vi "micron_ui.vi"() -> ()   [LabVIEW 2014]
uses:
  testing/Trace controls.ctl
  testing/probe_point.ctl
  cancellation/sq_control_params.ctl
  cancellation/decoupled_gain.ctl
  testing/mode_conrols.ctl
  testing/control_selector.ctl
  testing/stimulus.ctl
  testing/injection_point.ctl
  filtering/goal_loop_parms.ctl
  host/network_params.ctl
  cancellation/estimation_controls.ctl
  testing/flag_selector.ctl
  testing/status_flag.ctl
  testing/pose_selector.ctl
  testing/pose_source.ctl
  testing/pose_relative_to.ctl
  testing/log_event.ctl
  <vilib>/Platform/TimedLoop/XDataNode/timing_clust.ctl
  <vilib>/Platform/TimedLoop/XDataNode/nitl_modes.ctl
  <vilib>/Platform/TimedLoop/XDataNode/wakeup.ctl
  testing/ui_override_opts.ctl
  initialization/micron_globals.vi
  <vilib>/Utility/xml.llb/Read From XML File(array).vi
  <vilib>/Utility/xml.llb/Write to XML File(string).vi
  <vilib>/Platform/TimedLoop/XDataNode/XDataNode.xnode
  <vilib>/Platform/TimedLoop/XDataNode/XDNodeRunTimeDep.lvlib
panel:
  in  "Tab Control":T1(tab)
  in  "Goal filter A":T2={"Speedup max"=100.0, "Speedup thresh"=1500.0, "Speedup nonlin"=2.0, "Filters"=[{"Lower Fc"=0.05, "Lower Q"=0.62, "Scale factor"=3.0, "Upper Fc"=2.0, "Upper Q"=0.62, "V limit"=1000.0, "V limit range"=1000.0}, {"Lower Fc"=0.05, "Lower Q"=0.62, "Scale factor"=3.0, "Upper Fc"=2.0, "Upper Q"=0.62, "V limit"=1000.0, "V limit range"=1000.0}]} {"Filters"."V limit range" format="%_3p"; "Filters"."V limit" format="%_3p"; "Filters"."Upper Q" format="%_3f"; "Filters"."Upper Fc" format="%_3p"; "Filters"."Lower Q" format="%_3f"; "Filters"."Scale factor" format="%_3f"; "Filters"."Lower Fc" format="%_3p"; "Speedup nonlin" format="%_3p"; "Speedup thresh" format="%_3p"; "Speedup max" format="%_3p"}
  in  "Goal filter B":T2={"Speedup max"=10.0, "Speedup thresh"=750.0, "Speedup nonlin"=2.0, "Filters"=[{"Lower Fc"=1.5, "Lower Q"=0.62, "Scale factor"=1.0, "Upper Fc"=1.5, "Upper Q"=0.62, "V limit"=1000.0, "V limit range"=0.0}, {"Lower Fc"=1.5, "Lower Q"=0.62, "Scale factor"=1.0, "Upper Fc"=1.5, "Upper Q"=0.62, "V limit"=1000.0, "V limit range"=0.0}]} {"Filters"."V limit range" format="%_3p"; "Filters"."V limit" format="%_3p"; "Filters"."Upper Q" format="%_3f"; "Filters"."Upper Fc" format="%_3p"; "Filters"."Lower Q" format="%_3f"; "Filters"."Scale factor" format="%_3f"; "Filters"."Lower Fc" format="%_3p"; "Speedup nonlin" format="%_3p"; "Speedup thresh" format="%_3p"; "Speedup max" format="%_3p"}
  in  "Transition time":sgl=1.0
  in  "Cancellation":T3={"KP"={"XY"=0.5, "Rxy"=0.5, "Z"=0.2, "Rz"=0.1}, "KI"=0.0, "KD"={"XY"=-0.2, "Rxy"=0.0, "Z"=0.0, "Rz"=0.0}, "Max vel"=13.0, "Max acc"=2.0, "Int error limit"=3.0, "RCM gain"=1.0, "Bypass"=FALSE, "Degraded gain"=0.4} {"Degraded gain" min=0 max=1 step=0.1 format="%#_3p"; "RCM gain" min=0 max=1 step=0.1 format="%#_3p"; "KD"."Rz" min=-1 max=1 step=0.01 format="%#_3p"; "KD"."Rxy" min=-1 max=1 step=0.01 format="%#_3p"; "KD"."Z" min=-1 max=1 step=0.01 format="%#_3p"; "KD"."XY" min=-1 max=1 step=0.01 format="%#_3p"; "KI" min=0 max=1 step=0.01 format="%#_3p"; "KP"."Rz" min=-1 max=1 step=0.01 format="%#_3p"; "KP"."Rxy" min=-1 max=1 step=0.01 format="%#_3p"; "KP"."Z" min=-1 max=1 step=0.01 format="%#_3p"; "KP"."XY" min=-1 max=1 step=0.01 format="%#_3p"; "Max acc" format="%#_3p"}
  in  "Estimation":T5={"Link"={"Measure noise"=[4.0], "Process noise"=[15.0, 1.0], "Alt process noise"=[20.0], "Alt turnoff cycles"=20, "Innovation limit"=[inf], "Residue threshold"=20.0, "Enable"=TRUE}, "Handle"={"Measure noise"=[3.6, 0.00036], "Process noise"=[0.0, 0.0, 0.3, 0.0, 0.0006, 0.3, 1.0, 0.3, 0.3, 1.0], "State limits"=[], "Innovation limit"=[], "Prediction Lookahead"=1.5, "Enable"=TRUE}}
  in  "Manipulator disable":bool
  in  "Network":T6={"Remote Host"="192.168.1.3", "Send Status"=TRUE, "Send Port"=61557, "Recv Commands"=FALSE, "Recv Port"=61557}
  in  "Light enables":bool[](array[boolean])=[TRUE, TRUE, TRUE, TRUE, TRUE, TRUE]
  out "Trace display":T7(graph)
  out "Warning":bool
  out "Error":bool
  out "Status":T8[](array[typedef]) {"Timestamp" format="%<%.3X>T"}
  in  "Reference hold":bool
  in  "Pose selectors":T9[](array[typedef])
  in  "Recenter":bool
  out "RCM limit":bool
  out "Stall":bool[](array[boolean])
  out "Link lengths":sgl[](array[slide]) scale=-1.0..1.0
  out "Saturation":bool
  out "Speedup":sgl(slide) scale=1.0..50.0
  in  "Flag selectors":T12[](array[typedef])
  in  "Averaging":bool
  in  "Reset":bool
  out "Run/stop":bool
  in  "Trigger":bool
  in  "Trigger mode":bool
  in  "Calibration":bool=TRUE
  in  "Parameters":bool=TRUE
  in  "Controls":bool=TRUE
  in  "Load":bool
  in  "Configurations":i32(listbox)
  in  "Save":bool
  in  "Save as":bool
  in  "Config name":string="default"
  in  "Finder":bool=TRUE
  out "Position":sgl[](array[numeric]) format="%9.1f"
  in  "Stimulus":T14={"Type"=enum."Off", "Phase"=0.0, "Amplitude"=[0.0, 200.0, 0.0, 0.0, 0.0, 0.0], "Injection point"=enum."Total pose", "Closed loop"=TRUE, "Offset"=[0.0, 0.0, 0.0, 0.0, 0.0, 0.0], "Tip -> world"=TRUE, "Frequency"=1.0, "Length"=1.0} {"Length" min=0.0 max=100.0 step=100.0 format="%#_4p"; "Frequency" min=0.0 step=100.0 format="%#_4g"; "Offset" format="%#_3p"; "Amplitude" format="%#_3p"; "Phase" min=-180.0 max=360.0 step=100.0 format="%#.2f"}
  in  "Pedal selector":T16[](array[typedef])=[{"Selection"=enum."Right", "Mode"=enum."Never"}, {"Selection"=enum."Left", "Mode"=enum."Toggle"}, {"Selection"=enum."Right", "Mode"=enum."Toggle"}, {"Selection"=enum."Middle", "Mode"=enum."Pulse"}]
  out "Mode controls":T17={"Hold"=FALSE, "Cancellation"=TRUE, "Goal filter"=TRUE, "Trigger"=FALSE}
  in  "Decimate":i32=20 min=1 max=999 step=1
  in  "Trace path":path
  in  "Save trace":bool
  out "2D position":cluster{"X":sgl[], "Y":sgl[]}[](graph)
  in  "Trace controls":T18[](array[typedef])=[{"+ stim"=FALSE, "Relative"=FALSE, "Scale"=enum."1X", "Probe point"=enum."Position (tip)", "XYZ selector"={"Boolean"=FALSE, "Boolean 2"=FALSE, "Boolean 3"=FALSE}, "To tip"=FALSE}, {"+ stim"=FALSE, "Relative"=FALSE, "Scale"=enum."1X", "Probe point"=enum."Position (tip)", "XYZ selector"={"Boolean"=FALSE, "Boolean 2"=FALSE, "Boolean 3"=FALSE}, "To tip"=FALSE}, {"+ stim"=FALSE, "Relative"=FALSE, "Scale"=enum."1X", "Probe point"=enum."Position (tip)", "XYZ selector"={"Boolean"=FALSE, "Boolean 2"=FALSE, "Boolean 3"=FALSE}, "To tip"=FALSE}, {"+ stim"=FALSE, "Relative"=FALSE, "Scale"=enum."1X", "Probe point"=enum."Position (tip)", "XYZ selector"={"Boolean"=FALSE, "Boolean 2"=FALSE, "Boolean 3"=FALSE}, "To tip"=FALSE}]
  in  "stop":bool
  # "m  Micron interface"
  # "Triggering"
  # "One-shot"
  # "Continuous"
  # "Trace Display"
  # "Used for ASAP testing.  Not saved in config."
  # "Configuration Manager"
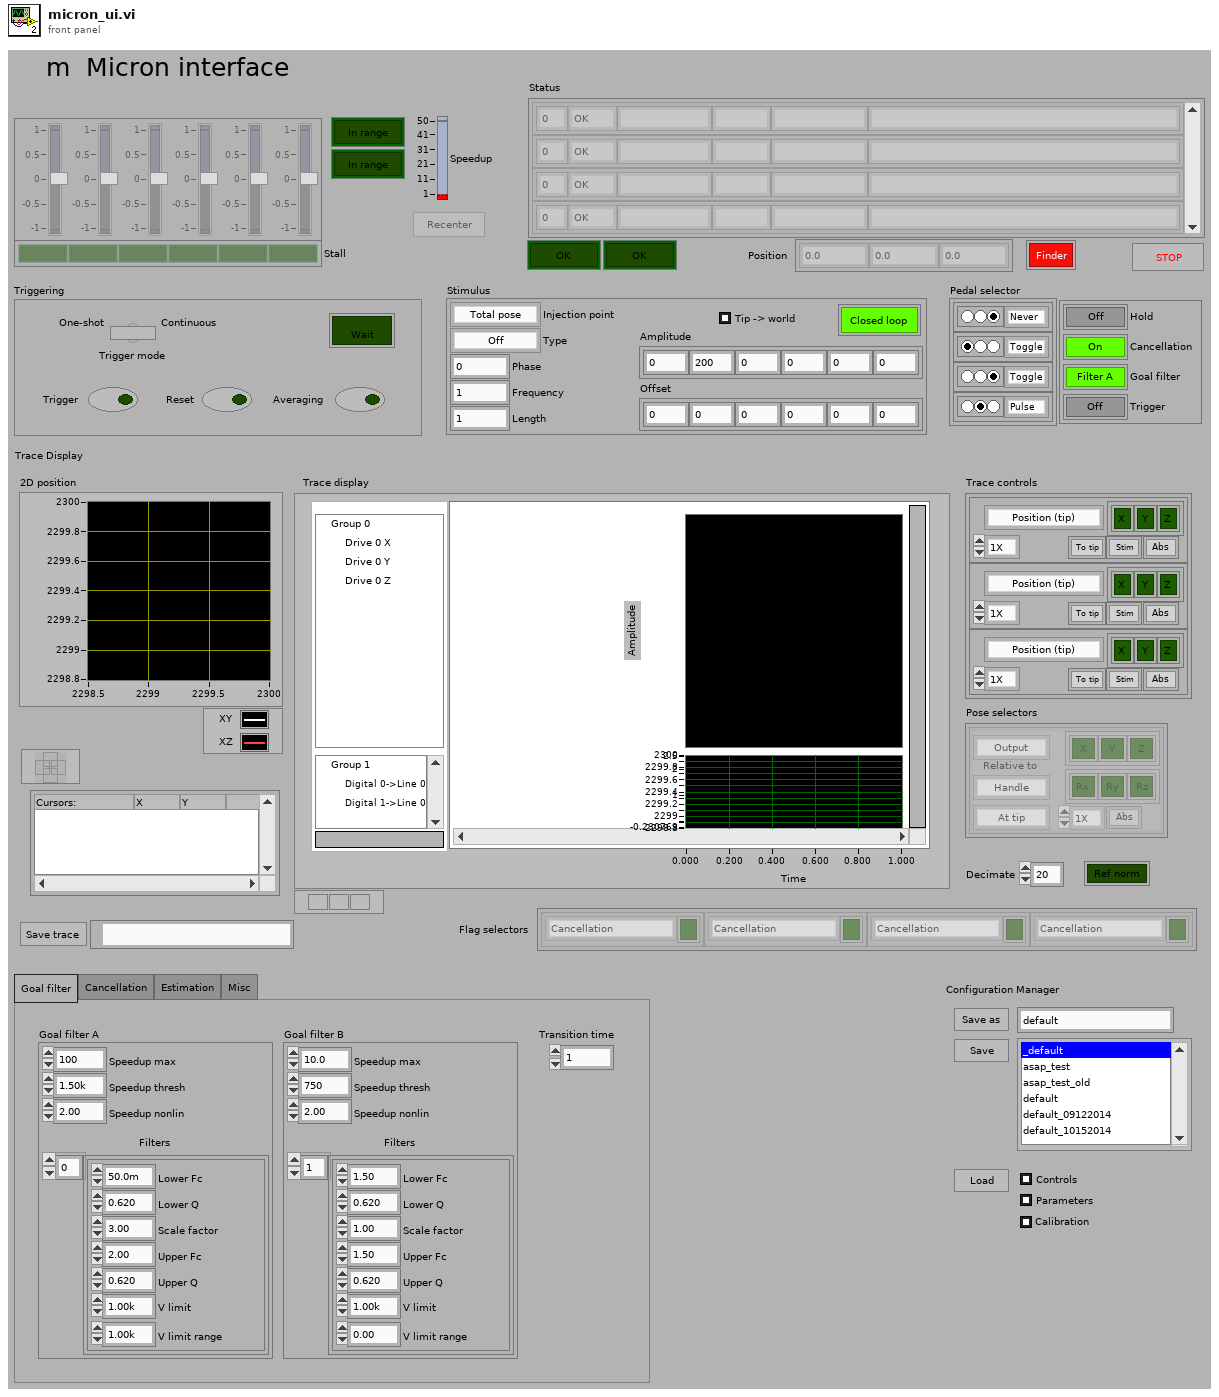
[diagram p1: front panel]
types:
  T1 = enum32{"Goal filter", "Cancellation", "Estimation", "Misc"}
  T2 = typedef "goal_loop_parms.ctl" = cluster{"Speedup max":sgl, "Speedup thresh":sgl, "Speedup nonlin":sgl, "Filters":cluster{"Lower Fc":sgl, "Lower Q":sgl, "Scale factor":sgl, "Upper Fc":sgl, "Upper Q":sgl, "V limit":sgl, "V limit range":sgl}[]}
  T3 = typedef "sq_control_params.ctl" = cluster{"KP":T4, "KI":sgl, "KD":T4, "Max vel":sgl, "Max acc":sgl, "Int error limit":sgl, "RCM gain":sgl, "Bypass":bool, "Degraded gain":sgl}
  T4 = typedef "decoupled_gain.ctl" = cluster{"XY":sgl, "Rxy":sgl, "Z":sgl, "Rz":sgl}
  T5 = typedef "estimation_controls.ctl" = cluster{"Link":cluster{"Measure noise":dbl[], "Process noise":dbl[], "Alt process noise":dbl[], "Alt turnoff cycles":i32, "Innovation limit":dbl[], "Residue threshold":dbl, "Enable":bool}, "Handle":cluster{"Measure noise":dbl[], "Process noise":dbl[], "State limits":dbl[], "Innovation limit":dbl[], "Prediction Lookahead":sgl, "Enable":bool}}
  T6 = typedef "network_params.ctl" = cluster{"Remote Host":string, "Send Status":bool, "Send Port":u16, "Recv Commands":bool, "Recv Port":u16}
  T7 = cluster{"Waveforms out":waveform(sgl)[], "Digital waveforms":digitalwaveform[]}
  T8 = typedef "log_event.ctl" = cluster{"Facility ID":i32, "Severity":enum16{"OK", "Debug", "Warn", "Error"}, "Timestamp":timestamp, "Facility":string, "State":string, "Message":string}
  T9 = typedef "pose_selector.ctl" = cluster{"Scale":enum16{"1X", "10X", "100X", "1KX", "10KX"}, "Source":T10, "XYZ selector":cluster{"Boolean":bool, "Boolean 2":bool, "Boolean 3":bool}, "RPY selector":cluster{"Boolean":bool, "Boolean 2":bool, "Boolean 3":bool}, "Relative to":T11, "Relative":bool, "Translate":enum16{"At tip", "At RCM", "At KC", "At origin"}}
  T10 = typedef "pose_source.ctl" = enum16{"Output", "Handle", "Handle KF", "Goal", "Absolute"}
  T11 = typedef "pose_relative_to.ctl" = enum16{"Output", "Handle", "Handle KF", "Goal", "Absolute", "Trace start"}
  T12 = typedef "flag_selector.ctl" = cluster{"Flag":T13, "Select":bool}
  T13 = typedef "status_flag.ctl" = enum16{"Cancellation", "Goal filter", "Valid position", "Goal saturation tip", "Goal saturation RCM", "Goal circle saturation", "Position saturation", "Output saturation", "Acceleration limiting", "Finished late", "Stimulus increasing", "Integral error saturation", "Velocity limiting", "Log warning", "Log error", "Link KF degraded"}
  T14 = typedef "stimulus.ctl" = cluster{"Type":enum16{"Off", "Step", "Sine", "Triangle", "Arbitrary"}, "Phase":dbl, "Amplitude":sgl[], "Injection point":T15, "Closed loop":bool, "Offset":sgl[], "Tip -> world":bool, "Frequency":dbl, "Length":dbl}
  T15 = typedef "injection_point.ctl" = enum16{"Total pose", "V limiter", "Goal ", "Link position", "KF link position", "Inverse kin", "Link goal", "Link error", "Controller", "Output", "Drive", "Light"}
  T16 = typedef "control_selector.ctl" = cluster{"Selection":enum32{"No Selection", "Left", "Middle", "Right"}, "Mode":enum16{"Up", "Down", "Toggle", "Pulse", "Always", "Never"}}
  T17 = typedef "mode_conrols.ctl" = cluster{"Hold":bool, "Cancellation":bool, "Goal filter":bool, "Trigger":bool}
  T18 = typedef "Trace controls.ctl" = cluster{"+ stim":bool, "Relative":bool, "Scale":enum16{"1X", "10X", "100X", "1KX", "10KX"}, "Probe point":T19, "XYZ selector":cluster{"Boolean":bool, "Boolean 2":bool, "Boolean 3":bool}, "To tip":bool}
  T19 = typedef "probe_point.ctl" = enum16{"Position (tip)", "Position (RCM)", "Null pos (tip)", "Null pos (RCM)", "V limiter (tip)", "V Limiter (RCM)", "Goal filter (tip)", "Goal filter (RCM)", "Goal force (tip)", "Goal force (RCM)", "Goal (tip)", "Goal (RCM)", "Link pos 0", "Link pos 1", "KF link pos 0", "KF link pos 1", "Link rate 0", "Link rate 1", "Link residue 0", "Link residue 1", "Link goal 0", "Link goal 1", "Rate limit 0", "Rate limit 1", "Link error 0", "Link error 1", "Controller 0", "Controller 1", "Output 0", "Output 1", "Drive 0", "Drive 1", "Stimulus 0", "Stimulus 1", "Trace data 0", "Trace data 1", "Analog data 0", "Analog data 1", "Status flags", "Light 0", "Light 1", "Light 2", "Light 3", "Light 4", "Light 5", "Goal origin", "Goal rotation 0", "Goal rotation 1", "Goal rotation 2", "Output origin", "Output rotation 0", "Output rotation 1", "Output rotation 2", "Handle origin", "Handle rotation 0", "Handle rotation 1", "Handle rotation 2", "Handle position", "Handle velocity", "Handle acceleration", "Handle angles", "Handle angle rates", "Handle pos residue", "Handle angle residue", "Trace length"}
  T20 = typedef "XDNodeRunTimeDep.lvlib/timing_clust.ctl" = cluster{"Expected End [f-1]":u64, "Actual End [f-1]":u64, "Finished Late? [f-1]":bool, "Expected End [i-1]":u64, "Actual End [i-1]":u64, "Finished Late? [i-1]":bool, "Expected Start [i]":u64, "Actual Start [i]":u64, "Expected Start [f]":u64, "Actual Start [f]":u64, "Source Name":string, "Structure Name":string, "Period":i64, "Deadline":i64, "Offset":i64, "Start":i64, "Priority":i32, "Timeout":i32, "Mode":T21, "Wakeup Reason":T22, "Error":errorcluster, "Source Type":string, "Secondary Source Type":string, "Global End Time":u64, "Global Start Time":u64, "Frame Duration":u64, "Iteration Duration":u64, "Assigned CPU":i32, "I/O Scan Engine Mode":u32}
  T21 = typedef "XDNodeRunTimeDep.lvlib/nitl_modes.ctl" = enum32{"No Change", "Process missed periods, maintain original phase", "Discard missed periods, maintain original phase", "Process missed periods, ignore original phase", "Discard missed periods, ignore original phase"}
  T22 = typedef "XDNodeRunTimeDep.lvlib/wakeup.ctl" = enum32{"Normal", "Aborted", "Asynchronous wakeup", "Timing source error", "Timed loop error", "Timeout"}
  T23 = typedef "micron_config.ctl" = cluster{"rt fifo":refnum<k33>, "Analog output task":refnum<k21>, "Analog output task 2":refnum<k21>, "Stimulus AO task":refnum<k21>, "Low-rate AIN task":refnum<k21>, "Pedal out task":refnum<k21>, "Pedal in task":refnum<k21>, "Loop timing source":string, "Relay out task":refnum<k21>, "Send UDP Conn":refnum<k16>, "Recv UDP Conn":refnum<k16>, "Host Addr":u32, "I2C interface":T24, "trace_start notifier":refnum<notifier>, "trace_done notifier":refnum<notifier>, "ASAP FIFO":refnum<k33>}
  T24 = typedef "i2c_interface.ctl" = cluster{"FPGA VI Reference":T25}
  T25 = typedef "fpga_reference.ctl" = refnum<k20>
  T26 = typedef "configuration.ctl" = cluster{"Calibration data":T27, "Block size":i32, "Tasks":cluster{"Analog Input":refnum<k21>, "Counters":refnum<k21>[], "Digital out":refnum<k21>}, "Light enables":bool[]}
  T27 = typedef "asap_calibration.ctl" = cluster{"T1":T28, "K1":T28, "T2":T28, "K2":T28, "Sensor LUT":sgl[][][][]}
  T28 = typedef "NI_Matrix.lvlib/RealMatrix.ctl" = dbl[][]
  T29 = enum8{"Enabled", "Disabled", "Disabled and Grayed Out"}
  T30 = typedef "Micron params.ctl" = cluster{"Stimulus":T14, "Goal Filter A":T2, "Mode controls":T17, "Manipulator type":enum16{"Current piezo", "Voltage piezo"}, "Manipulator calibration":T31, "Network":T6, "Goal Filter B":T2, "Cancellation":T3, "Transition time":sgl, "Estimation":T5}
  T31 = typedef "manipulator_cal.ctl" = cluster{"Tool offsets":sgl[][], "Handle light calibration":T32, "Base pivots":sgl[][], "Output pivots":sgl[][], "Length center":sgl, "Workspace height":sgl[], "Workspace diameter":sgl[], "Stack travel":sgl, "Saturation pos":sgl, "Inverse filters":cluster{"filter structure":enum32{"IIR 2nd Order", "IIR 4th Order"}, "Reverse Coefficients":dbl[], "Forward Coefficients":dbl[]}[], "Strut length":sgl, "Tip light calibration":T32}
  T32 = typedef "probe_calibration.ctl" = sgl[][]
  T33 = typedef "ui_override_opts.ctl" = cluster{"Triggering":bool, "Parameters":bool, "Stimulus":bool, "Calibration":bool, "Modes":bool}
  T34 = enum16{"Up", "Down", "Toggle", "Pulse", "Always", "Never"}
  T35 = cluster{"Finder":bool, "Trigger mode":bool, "Pedal selector":T16[], "Decimate":i32, "Trace controls":T18[], "Flag selectors":T12[], "Pose selectors":T9[]}
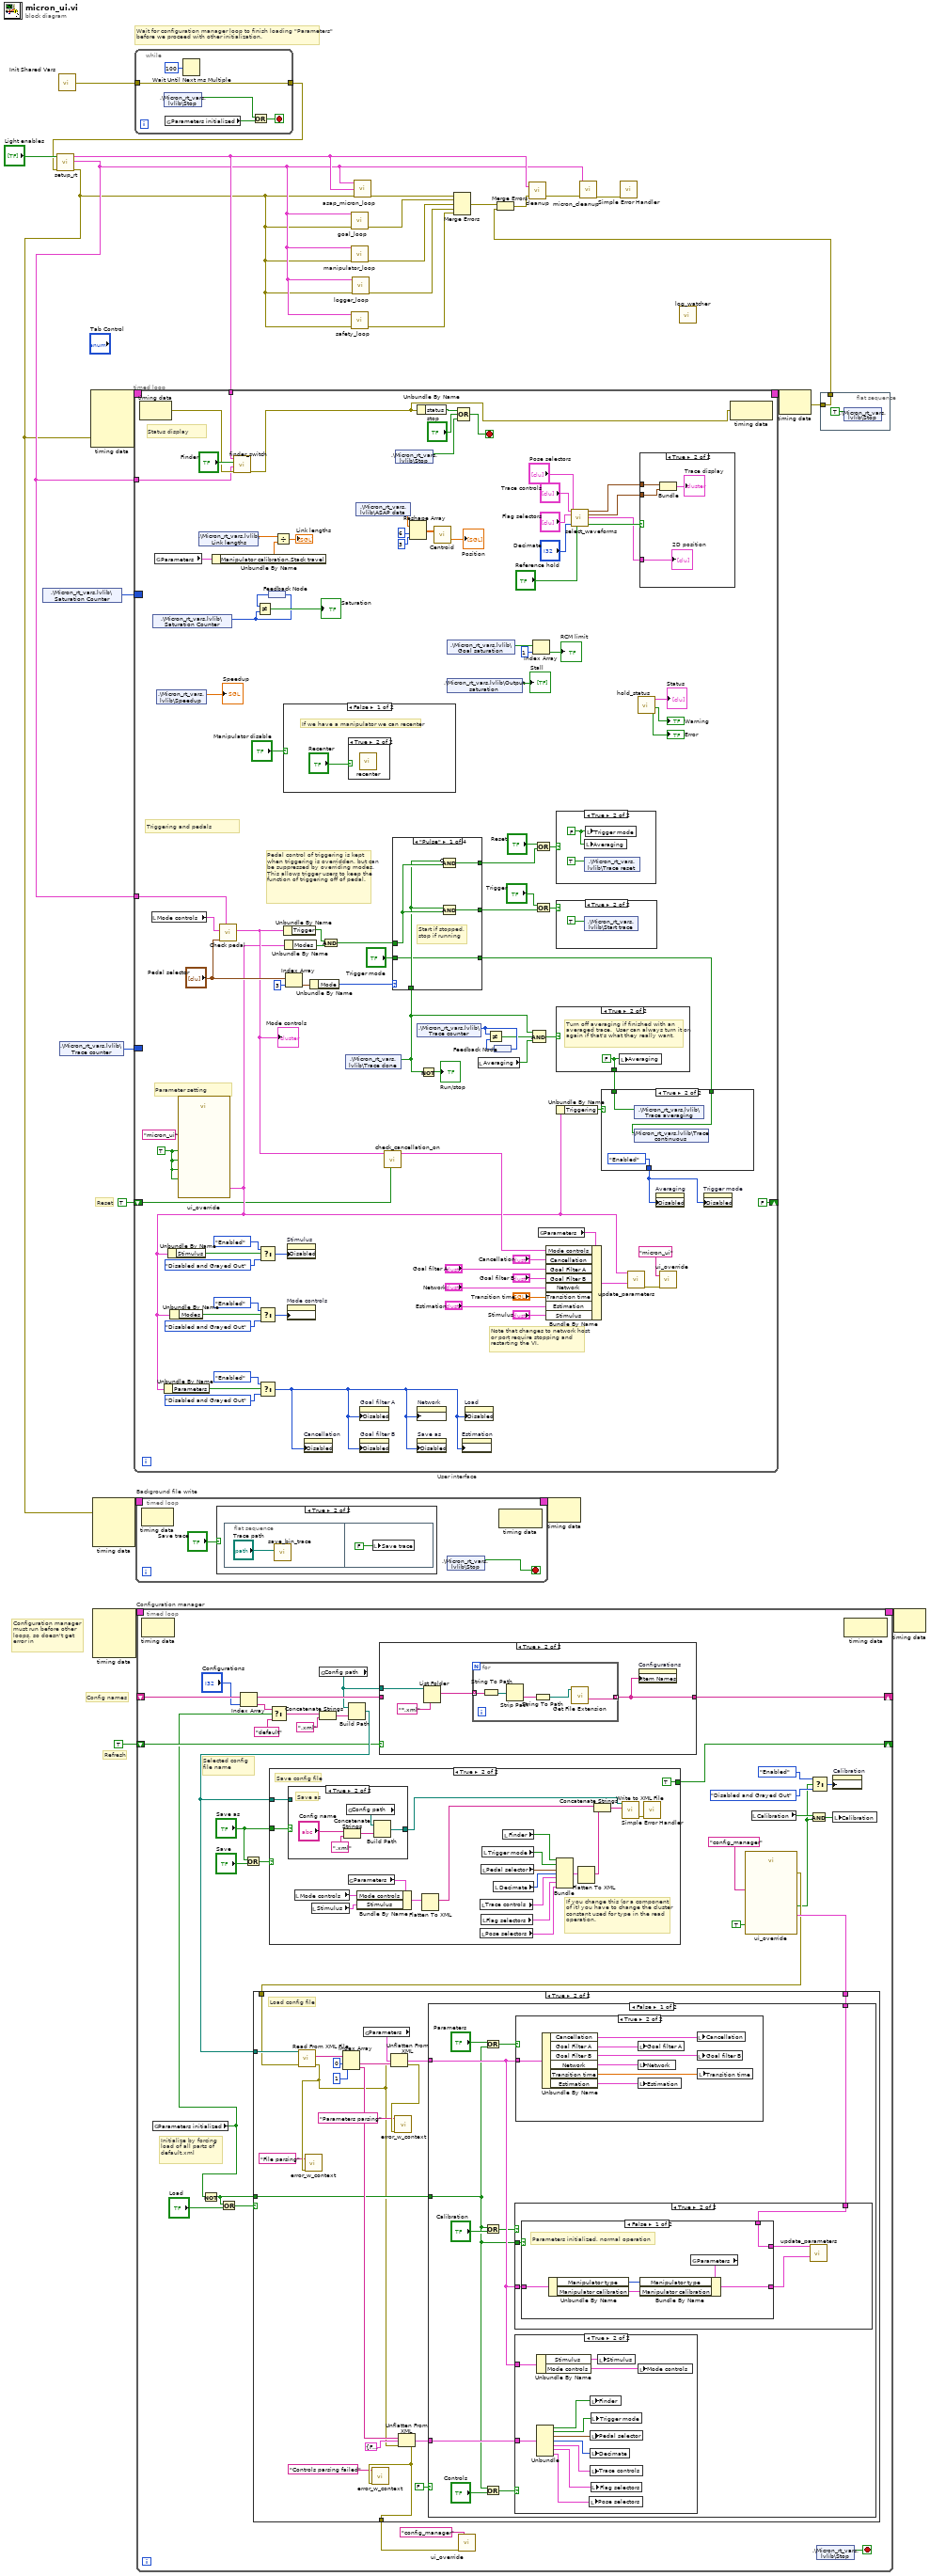
[diagram p0: block diagram]
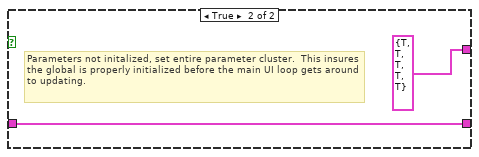
[diagram p4: hidden frame]
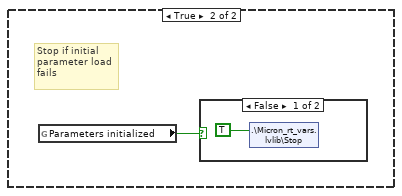
[diagram p7: hidden frame]
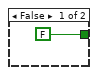
[diagram p9: hidden frame]
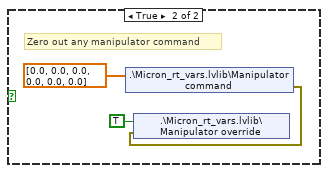
[diagram p14: hidden frame]
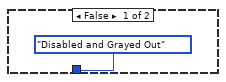
[diagram p15: hidden frame]
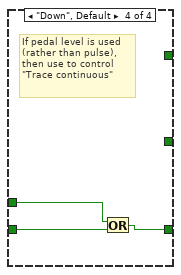
[diagram p18: hidden frame]
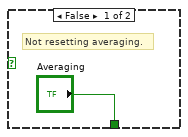
[diagram p19: hidden frame]
diagram:
  # "Reset"
  # "Configuration manager \nmust run before other\nloops, so doesn't get\nerror in"
  # "Wait for configuration manager loop to finish loading \"Parameters\" before we proceed with other initialization."
  # "Config names"
  # "Refresh"
  n1 = shared-variable ".\\Micron_rt_vars.lvlib\\Saturation Counter"() -> (w19:u32)  [unwired: 2 out]
  n2 = call "Init Shared Vars.vi"() -> ("error out"=w15:errorcluster)  [unwired: 1 in]
  n3 = shared-variable ".\\Micron_rt_vars.lvlib\\Trace counter"() -> (w13:u32)  [unwired: 2 out]
  n4 = node-c288() -> (w17:T20)  [unwired: 4 out]
  n5 = while {
    tunnel: w15 -> [w32]
    tunnel: [w32] -> w14
    stop <- w30 stop-if-true
    n6 = shared-variable ".\\Micron_rt_vars.lvlib\\Stop"() -> (w28:bool)  [unwired: 2 out]
    n7 = global read "micron_globals.vi" "Parameters initialized"() -> (w29:bool)
    n8 = Wait Until Next ms Multiple(millisecond multiple=u32 100) -> ()  [unwired: 1 out]
    n9 = Or(x=w28, y=w29) -> (x .or. y?=w30:bool)
  }
  n10 = call "setup_rt.vi"("error in"=w14, "Light enables"="Light enables") -> ("error out"=w9:errorcluster, "Micron config"=w11:T23, "ASAP Config"=w21:T26)  [unwired: 5 out]
  n11 = node-c288(w9) -> (w27:T20)  [unwired: 4 out]
  n12 = node-c288(w9) -> (w24:T20)  [unwired: 3 out]
  n13 = timed-loop "User interface" {
    timing: w27 -> [_]
    timing-out: [_] -> w26
    tunnel: w21 -> [w122]
    tunnel: w11 -> [w111]
    border: w13 -> [_]
    border: w19 -> [_]
    tunnel: w11 -> [w78]
    shift-right: [FALSE ("Reset")] -> _
    shift-left: TRUE ("Reset") -> [w36]
    stop <- w127 stop-if-true
    w73 = TRUE ("Parameters")
    # "Pedal control of triggering is kept when triggering is overridden, but can be suppressed by overriding modes.  This allows trigger users to keep the function of triggering off of pedal."
    # "Note that changes to network host or port require stopping and restarting the VI."
    # "Status display"
    # "Parameter setting"
    # "Triggering and pedals"
    n14 = node-c288() -> (w80:errorcluster)  [unwired: 1 out]
    n15 = local read "Mode controls"() -> (w112:T17)
    n16 = shared-variable ".\\Micron_rt_vars.lvlib\\Saturation Counter"() -> (w119:u32)  [unwired: 2 out]
    n17 = global read "micron_globals.vi" "Parameters"() -> (w110:T30)
    n18 = shared-variable ".\\Micron_rt_vars.lvlib\\Speedup"() -> (→"Speedup":sgl)  [unwired: 2 out]
    n19 = call "ui_override.vi"("Triggering"=w73, "VI name"="micron_ui", "Parameters"=w73, "Stimulus"=w73, "Modes"=w73) -> ("Override"=w40:T33)  [unwired: 8 in, 2 out]
    n20 = Unbundle By Name(w40) -> ("Parameters"=w72:bool)
    n21 = Unbundle By Name(w40) -> ("Stimulus"=w67:bool)
    n22 = Unbundle By Name(w40) -> ("Modes"=w65:bool)
    n23 = shared-variable ".\\Micron_rt_vars.lvlib\\Link lengths"() -> (w109:sgl[])  [unwired: 2 out]
    n24 = Unbundle By Name(w110) -> ("Manipulator calibration.Stack travel"=w108:sgl)
    n25 = call "Check pedal.vi"("Micron config"=w111, "Pedal selector"="Pedal selector", "Mode controls"=w112) -> ("New mode controls"=w44:T17)  [unwired: 8 out]
    "Mode controls" <- w44
    n26 = call "finder_switch.vi"("error in"=w80, "Micron config"=w78, "Finder"="Finder", "Configuration"=w122) -> ("error out"=w79:errorcluster)  [unwired: 5 out]
    n27 = Select(t=T29."Enabled" ("Disabled"), s=w67, f=T29."Disabled and Grayed Out" ("Disabled")) -> (s? t:f=w66:T29)
    n28 = Select(t=T29."Enabled" ("Disabled"), s=w65, f=T29."Disabled and Grayed Out" ("Disabled")) -> (s? t:f=w62:T29)
    n29 = Select(t=T29."Enabled" ("Disabled"), s=w72, f=T29."Disabled and Grayed Out" ("Disabled")) -> (s? t:f=w49:T29)
    n30 = feedback-in #1(w119) -> ()
    n31 = feedback #1() -> (w121:u32)
    n32 = Not Equal?(x=w121, y=w119) -> (x != y?=→"Saturation":bool)
    n33 = Divide(x=w109, y=w108) -> (x/y=→"Link lengths":sgl[])
    n34 = case shown="False" "Manipulator disable" {
      frame False {
        # "If we have a manipulator we can recenter"
        n35 = case shown="True" "Recenter" {
          frame False {
          }
          frame True {
            n36 = call "recenter.vi"() -> ()  [unwired: 1 in]
          }
        }
      }
      frame True {
        # "Zero out any manipulator command"
        n37 = shared-variable ".\\Micron_rt_vars.lvlib\\Manipulator command"(sgl[] [0.0, 0.0, 0.0, 0.0, 0.0, 0.0] ("Manipulator command")) -> (error out=w131:errorcluster)  [unwired: 1 in]
        n38 = shared-variable ".\\Micron_rt_vars.lvlib\\Manipulator override"(TRUE ("Manipulator override"), error in=w131) -> ()  [unwired: 1 out]
      }
    }
    n39 = Unbundle By Name(w44) -> ("Trigger"=w38:bool)
    n40 = Unbundle By Name(w40) -> ("Modes"=w39:bool)
    n41 = Index Array(array="Pedal selector", index=3) -> (element=w83:T16)
    n42 = property on="Stimulus" class="Clust (strict)"("Disabled"=w66) -> ()  [unwired: 2 in, 2 out]
    n43 = property on="Mode controls" class="Clust (strict)"("DisabledEnum"=w62) -> ()  [unwired: 2 in, 2 out]
    n44 = property on="Cancellation" class="Clust (strict)"("Disabled"=w49) -> ()  [unwired: 2 in, 2 out]
    n45 = Unbundle By Name(w83) -> ("Mode"=w81:T34)
    n46 = And(x=w38, y=w39) -> (x .and. y?=w37:bool)
    n47 = shared-variable ".\\Micron_rt_vars.lvlib\\Trace done"() -> (w86:bool)  [unwired: 2 out]
    n48 = shared-variable ".\\Micron_rt_vars.lvlib\\ASAP data"() -> (w105:sgl[])  [unwired: 2 out]
    n49 = property on="Goal filter A" class="Clust (strict)"("Disabled"=w49) -> ()  [unwired: 2 in, 2 out]
    n50 = property on="Goal filter B" class="Clust (strict)"("Disabled"=w49) -> ()  [unwired: 2 in, 2 out]
    n51 = call "check_cancellation_on.vi"("Reset"=w36, "Mode controls in"=w44) -> ("Mode controls out"=w54:T17)  [unwired: 9 in]
    n52 = case shown="\"Pulse\"" w81 {
      tunnel: [w141 _ _ _] -> w114
      tunnel: [w140 _ _ _] -> w113
      tunnel: w37 -> [w139 _ _ w144]
      tunnel: w86 -> [w138 _ _ _]
      tunnel: [w137 w142 w143 w146] -> w77
      tunnel: "Trigger mode" -> [w137 w142 w143 w145]
      frame "Pulse" {
        # "Start if stopped, stop if running"
        n53 = Compound Arithmetic op=AND(invert w138, w139) -> (w141:bool)
        n54 = Compound Arithmetic op=AND(w138, w139) -> (w140:bool)
      }
      frame "Always" {
        # "Don't actually force continuous, since it may be confusing, and they can always do that explicitly with \"Trigger mode\""
      }
      frame "Never" {
      }
      frame "Down", Default {
        # "If pedal level is used (rather than pulse), then use to control \"Trace continuous\""
        n55 = Or(x=w144, y=w145) -> (x .or. y?=w146:bool)
      }
    }
    n56 = shared-variable ".\\Micron_rt_vars.lvlib\\Stop"() -> (w125:bool)  [unwired: 2 out]
    n57 = Reshape Array(w105, 6 ("dimension size"), 3 ("dimension size")) -> (w104:sgl[][])
    n58 = Unbundle By Name(w79) -> ("status"=w128:bool)
    n59 = shared-variable ".\\Micron_rt_vars.lvlib\\Trace counter"() -> (w100:u32)  [unwired: 2 out]
    n60 = property on="Network" class="Clust (strict)"("DisabledEnum"=w49) -> ()  [unwired: 2 in, 2 out]
    n61 = property on="Save as" class="Bool"("Disabled"=w49) -> ()  [unwired: 2 in, 2 out]
    n62 = Not(x=w86) -> (.not. x?=→"Run/stop":bool)
    n63 = call "Centroid.vi"("Points"=w104) -> ("Centroid"=→"Position":sgl[])  [unwired: 1 in, 1 out]
    n64 = shared-variable ".\\Micron_rt_vars.lvlib\\Goal saturation"() -> (w96:bool[])  [unwired: 2 out]
    n65 = shared-variable ".\\Micron_rt_vars.lvlib\\Output saturation"() -> (→"Stall":bool[])  [unwired: 2 out]
    n66 = Compound Arithmetic op=OR(w128, "stop", w125) -> (w127:bool)
    n67 = property on="Estimation" class="Clust (strict)"("DisabledEnum"=w49) -> ()  [unwired: 2 in, 2 out]
    n68 = property on="Load" class="Bool"("Disabled"=w49) -> ()  [unwired: 2 in, 2 out]
    n69 = local read "Averaging"() -> (w98:bool)
    n70 = feedback-in #2(w100) -> ()
    n71 = feedback #2() -> (w101:u32)
    n72 = Not Equal?(x=w100, y=w101) -> (x != y?=w99:bool)
    n73 = Index Array(array=w96, index=1) -> (element=→"RCM limit":bool)
    n74 = Compound Arithmetic op=AND(w86, w99, w98) -> (w102:bool)
    n75 = Or(x="Reset", y=w114) -> (x .or. y?=w115:bool)
    n76 = Or(x="Trigger", y=w113) -> (x .or. y?=w103:bool)
    n77 = global read "micron_globals.vi" "Parameters"() -> (w55:T30)
    n78 = Bundle By Name(cluster=w55, "Mode controls"=w54, "Cancellation"="Cancellation", "Goal Filter A"="Goal filter A", "Goal Filter B"="Goal filter B", "Network"="Network", "Transition time"="Transition time", "Estimation"="Estimation", "Stimulus"="Stimulus") -> (w53:T30)
    n79 = Unbundle By Name(w40) -> ("Triggering"=w75:bool)
    n80 = case shown="True" w115 {
      frame False {
      }
      frame True {
        w149 = FALSE ("Trigger mode")
        n81 = local write "Averaging"(w149) -> ()
        n82 = shared-variable ".\\Micron_rt_vars.lvlib\\Trace reset"(TRUE ("Start trace")) -> ()  [unwired: 2 out]
        n83 = local write "Trigger mode"(w149) -> ()
      }
    }
    n84 = case shown="True" w103 {
      frame False {
      }
      frame True {
        n85 = shared-variable ".\\Micron_rt_vars.lvlib\\Start trace"(TRUE ("Start trace")) -> ()  [unwired: 2 out]
      }
    }
    n86 = case shown="True" w102 {
      tunnel: ["Averaging" w148] -> w76
      frame False {
        # "Not resetting averaging."
      }
      frame True {
        w148 = FALSE ("Averaging")
        # "Turn off averaging if finished with an averaged trace.  User can always turn it on again if that's what they really want."
        n87 = local write "Averaging"(w148) -> ()
      }
    }
    n88 = call "select_waveforms.vi"("Trace controls"="Trace controls", "Flag selectors"="Flag selectors", "Pose selectors"="Pose selectors", "Decimate"="Decimate", "Reference hold"="Reference hold") -> ("Waveforms out"=w90:waveform(sgl)[], "Digital waveforms"=w89:digitalwaveform[], "XY views"=w91:cluster{"X":sgl[], "Y":sgl[]}[], "New data"=w92:bool)  [unwired: 7 in]
    n89 = case shown="True" w75 {
      tunnel: w77 -> [_ w136]
      tunnel: w76 -> [_ w135]
      tunnel: [T29."Disabled and Grayed Out" ("Disabled") T29."Enabled" ("Disabled")] -> w61
      frame False {
      }
      frame True {
        n90 = shared-variable ".\\Micron_rt_vars.lvlib\\Trace averaging"(w135) -> ()  [unwired: 2 out]
        n91 = shared-variable ".\\Micron_rt_vars.lvlib\\Trace continuous"(w136) -> ()  [unwired: 2 out]
      }
    }
    n92 = call "update_parameters.vi"("Modify"=w40, "Parameters"=w53) -> ("error out"=w50:errorcluster)  [unwired: 12 in, 1 out]
    n93 = call "hold_status.vi"() -> ("Error"=→"Error":bool, "Warning"=→"Warning":bool, "Hold status"=→"Status":T8[])  [unwired: 9 in]
    n94 = case shown="True" w92 {
      tunnel: w90 -> [_ w154]
      tunnel: w91 -> [_ w155]
      tunnel: w89 -> [_ w153]
      frame False {
      }
      frame True {
        n95 = Bundle("Waveforms out"=w154, "Digital waveforms"=w153) -> (→"Trace display":T7)  [unwired: 1 in]
        "2D position" <- w155
      }
    }
    n96 = property on="Averaging" class="Bool (strict)"("Disabled"=w61) -> ()  [unwired: 2 in, 2 out]
    n97 = call "ui_override.vi"("VI name"="micron_ui", "error in"=w50) -> ()  [unwired: 11 in, 3 out]
    n98 = property on="Trigger mode" class="Bool (strict)"("Disabled"=w61) -> ()  [unwired: 2 in, 2 out]
    n99 = node-c288(w79) -> ()  [unwired: 1 out]
  }
  n100 = timed-loop "Background file write" {
    timing: w24 -> [_]
    timing-out: [_] -> w23
    stop <- w161 stop-if-true
    n101 = node-c288() -> ()  [unwired: 2 out]
    n102 = case shown="True" "Save trace" {
      frame False {
      }
      frame True {
        n103 = flat-sequence {
          frame #0 {
            n104 = call "save_bin_trace.vi"("File path"="Trace path") -> ()  [unwired: 1 in, 10 out]
          }
          frame #1 {
            n105 = local write "Save trace"(FALSE ("Save trace")) -> ()
          }
        }
      }
    }
    n106 = shared-variable ".\\Micron_rt_vars.lvlib\\Stop"() -> (w161:bool)  [unwired: 2 out]
    n107 = node-c288() -> ()  [unwired: 2 out]
  }
  n108 = timed-loop "Configuration manager" {
    shift-right: [w191] -> _
    shift-left: TRUE -> [w188]
    shift-right: [w198] -> _
    shift-left: _ -> [w197]
    timing: w17 -> [_]
    timing-out: [_] -> w16
    stop <- w187 stop-if-true
    # "Initialize by forcing load of all parts of default.xml"
    # "Selected config file name"
    n109 = node-c288() -> ()  [unwired: 2 out]
    n110 = global read "micron_globals.vi" "Parameters initialized"() -> (w180:bool)
    n111 = Not(x=w180) -> (.not. x?=w179:bool)
    n112 = Or(x=w179, y="Load") -> (x .or. y?=w184:bool)
    n113 = Index Array(array=w197, index="Configurations") -> (element=w183:string)
    n114 = Or(x="Save as", y="Save") -> (x .or. y?=w190:bool)
    n115 = Select(t=w183, s=w180, f="default") -> (s? t:f=w182:string)
    n116 = global read "micron_globals.vi" "Config path"() -> (w186:path)
    n117 = Concatenate Strings(w182, ".xml" ("string")) -> (w194:string)
    n118 = Build Path(base path=w186, name or relative path=w194) -> (appended path=w189:path)
    n119 = case shown="True" w190 {
      tunnel: "Save as" -> [_ w284]
      tunnel: w189 -> [_ w283]
      tunnel: [FALSE TRUE] -> w191
      frame False {
      }
      frame True {
        # "If you change this (or a component\nof it) you have to change the cluster constant used for type in the read operation."
        # "Save config file"
        n120 = case shown="True" w284 {
          tunnel: [w286 w288] -> w282
          tunnel: w283 -> [w286 _]
          frame False {
          }
          frame True {
            # "Save as"
            n121 = Concatenate Strings("Config name", ".xml" ("string")) -> (w291:string)
            n122 = global read "micron_globals.vi" "Config path"() -> (w287:path)
            n123 = Build Path(base path=w287, name or relative path=w291) -> (appended path=w288:path)
          }
        }
        n124 = local read "Mode controls"() -> (w270:T17)
        n125 = local read "Stimulus"() -> (w268:T14)
        n126 = global read "micron_globals.vi" "Parameters"() -> (w271:T30)
        n127 = Bundle By Name(cluster=w271, "Mode controls"=w270, "Stimulus"=w268) -> (w269:T30)
        n128 = Flatten To XML(anything=w269) -> (xml string=w273:string)
        n129 = local read "Trace controls"() -> (w280:T18[])
        n130 = local read "Pose selectors"() -> (w266:T9[])
        n131 = local read "Pedal selector"() -> (w278:T16[])
        n132 = local read "Flag selectors"() -> (w267:T12[])
        n133 = local read "Trigger mode"() -> (w277:bool)
        n134 = local read "Decimate"() -> (w279:i32)
        n135 = local read "Finder"() -> (w276:bool)
        n136 = Bundle("Finder"=w276, "Trigger mode"=w277, "Pedal selector"=w278, "Decimate"=w279, "Trace controls"=w280, "Flag selectors"=w267, "Pose selectors"=w266) -> (w275:T35)  [unwired: 1 out]
        n137 = Flatten To XML(anything=w275) -> (xml string=w272:string)
        n138 = Concatenate Strings(w273, w272) -> (w274:string)
        n139 = call-poly <vilib>:"Write to XML File.vi"("XML Input"=w274, "XML File Path"=w282) -> ("error out"=w285:errorcluster)  [unwired: 3 in, 6 out]
        n140 = call <vilib>:"Simple Error Handler.vi"("error in (no error)"=w285) -> ()  [unwired: 2 in, 7 out]
      }
    }
    n141 = case shown="True" w188 {
      tunnel: [w292 w294] -> w198
      tunnel: w197 -> [w292 _]
      tunnel: w186 -> [_ w293]
      frame False {
      }
      frame True {
        n142 = List Folder(path=w293, pattern="*.xml") -> (filenames=w296:string[])  [unwired: 1 in, 4 out]
        n143 = for {
          tunnel: w296 -> [w301] mode=indexing
          tunnel: [w297] -> w294 mode=indexing
          n144 = String To Path(string=w301) -> (path=w300:path)
          n145 = Strip Path(path=w300) -> (name=w299:string)  [unwired: 1 out]
          n146 = String To Path(string=w299) -> (path=w298:path)
          n147 = call <vilib>:"Get File Extension.vi"("file"=w298) -> ("filename without extension"=w297:string)  [unwired: 1 in, 9 out]
        }
        n148 = property on="Configurations" class="LstBox (strict)"("Item Names"=w294) -> ()  [unwired: 2 in, 2 out]
      }
    }
    n149 = call "ui_override.vi"("VI name"="config_manager", "Calibration"=TRUE ("Parameters")) -> ("Override"=w176:T33, "Got all"=w167:bool, "error out"=w171:errorcluster)  [unwired: 11 in]
    n150 = case shown="True" w184 {
      tunnel: w189 -> [_ w221]
      tunnel: w179 -> [_ w212]
      tunnel: w176 -> [_ w211]
      tunnel: w171 -> [w201 w210]
      tunnel: [w201 w207] -> w170
      frame False {
      }
      frame True {
        # "Load config file"
        n151 = call-poly <vilib>:"Read From XML File.vi"("error in (no error)"=w210, "XML File Path"=w221) -> ("error out"=w203:errorcluster, "XML Elements"=w217:string[])  [unwired: 8 out]
        n152 = call "error_w_context.vi"("error in (no error)"=w203, "error source"="File parsing") -> ()  [unwired: 10 in]
        n153 = Index Array(array=w217, index #1=0 ("index"), index #2=1 ("index")) -> (element #1=w220:string, element #2=w214:string)
        n154 = global read "micron_globals.vi" "Parameters"() -> (w216:T30)
        n155 = Unflatten From XML(xml string=w220, type=w216, error in (no error)=w203) -> (value=w218:T30, error out=w205:errorcluster)
        n156 = call "error_w_context.vi"("error in (no error)"=w205, "error source"="Parameters parsing" ("error source (\" \")")) -> ()  [unwired: 10 in]
        n157 = Unflatten From XML(xml string=w214, type=T35 {"Finder"=FALSE, "Trigger mode"=FALSE, "Pedal selector"=[], "Decimate"=0, "Trace controls"=[], "Flag selectors"=[], "Pose selectors"=[]} ("output cluster"), error in (no error)=w203) -> (value=w213:T35, error out=w207:errorcluster)
        n158 = call "error_w_context.vi"("error in (no error)"=w207, "error source"="Controls parsing failed" ("error source (\" \")")) -> ()  [unwired: 10 in]
        n159 = case shown="False" FALSE {
          tunnel: w218 -> [w230 _]
          tunnel: w213 -> [w231 _]
          tunnel: w212 -> [w223 _]
          tunnel: w211 -> [w222 _]
          frame False {
            n160 = Or(x="Parameters", y=w223) -> (x .or. y?=w229:bool)
            n161 = Or(x=w223, y="Calibration") -> (x .or. y?=w226:bool)
            n162 = Or(x=w223, y="Controls") -> (x .or. y?=w225:bool)
            n163 = case shown="True" w226 {
              tunnel: w230 -> [_ w236]
              tunnel: w223 -> [_ w234]
              tunnel: w222 -> [_ w232]
              frame False {
              }
              frame True {
                n164 = case shown="False" w234 {
                  tunnel: w236 -> [w242 w244]
                  tunnel: [w241 w244] -> w235
                  tunnel: [w237 T33 {"Triggering"=TRUE, "Parameters"=TRUE, "Stimulus"=TRUE, "Calibration"=TRUE, "Modes"=TRUE} ("Override")] -> w233
                  tunnel: w232 -> [w237 _]
                  frame False {
                    # "Parameters initialized, normal operation"
                    n165 = Unbundle By Name(w242) -> ("Manipulator type"=w239:enum16{"Current piezo", "Voltage piezo"}, "Manipulator calibration"=w238:T31)
                    n166 = global read "micron_globals.vi" "Parameters"() -> (w240:T30)
                    n167 = Bundle By Name(cluster=w240, "Manipulator type"=w239, "Manipulator calibration"=w238) -> (w241:T30)
                  }
                  frame True {
                    # "Parameters not initalized, set entire parameter cluster.  This insures the global is properly initialized before the main UI loop gets around to updating."
                  }
                }
                n168 = call "update_parameters.vi"("Modify"=w233, "Parameters"=w235) -> ()  [unwired: 12 in, 2 out]
              }
            }
            n169 = case shown="True" w225 {
              tunnel: w231 -> [_ w260]
              tunnel: w230 -> [_ w259]
              frame False {
              }
              frame True {
                n170 = Unbundle By Name(w259) -> ("Stimulus"=w257:T14, "Mode controls"=w258:T17)
                n171 = Unbundle(w260) -> ("Finder"=w262:bool, "Trigger mode"=w261:bool, "Pedal selector"=w256:T16[], "Decimate"=w255:i32, "Trace controls"=w254:T18[], "Flag selectors"=w253:T12[], "Pose selectors"=w252:T9[])
                n172 = local write "Pose selectors"(w252) -> ()
                n173 = local write "Finder"(w262) -> ()
                n174 = local write "Pedal selector"(w256) -> ()
                n175 = local write "Decimate"(w255) -> ()
                n176 = local write "Trace controls"(w254) -> ()
                n177 = local write "Trigger mode"(w261) -> ()
                n178 = local write "Flag selectors"(w253) -> ()
                n179 = local write "Stimulus"(w257) -> ()
                n180 = local write "Mode controls"(w258) -> ()
              }
            }
            n181 = case shown="True" w229 {
              tunnel: w230 -> [_ w248]
              frame False {
              }
              frame True {
                n182 = Unbundle By Name(w248) -> ("Cancellation"=w250:T3, "Goal Filter A"=w249:T2, "Goal Filter B"=w251:T2, "Network"=w247:T6, "Transition time"=w246:sgl, "Estimation"=w245:T5)
                n183 = local write "Goal filter A"(w249) -> ()
                n184 = local write "Network"(w247) -> ()
                n185 = local write "Estimation"(w245) -> ()
                n186 = local write "Cancellation"(w250) -> ()
                n187 = local write "Goal filter B"(w251) -> ()
                n188 = local write "Transition time"(w246) -> ()
              }
            }
          }
          frame True {
            # "Stop if initial\nparameter load\nfails"
            n189 = global read "micron_globals.vi" "Parameters initialized"() -> (w263:bool)
            n190 = case shown="False" w263 {
              frame False {
                n191 = shared-variable ".\\Micron_rt_vars.lvlib\\Stop"(TRUE ("stop - RT")) -> ()  [unwired: 2 out]
              }
              frame True {
              }
            }
          }
        }
      }
    }
    n192 = call "ui_override.vi"("VI name"="config_manager", "error in"=w170) -> ()  [unwired: 11 in, 3 out]
    n193 = local read "Calibration"() -> (w168:bool)
    n194 = And(x=w168, y=w167) -> (x .and. y?=w169:bool)
    n195 = Select(t=T29."Enabled" ("Disabled"), s=w167, f=T29."Disabled and Grayed Out" ("Disabled")) -> (s? t:f=w173:T29)
    n196 = shared-variable ".\\Micron_rt_vars.lvlib\\Stop"() -> (w187:bool)  [unwired: 2 out]
    n197 = property on="Calibration" class="Bool (strict)"("DisabledEnum"=w173) -> ()  [unwired: 2 in, 2 out]
    n198 = local write "Calibration"(w169) -> ()
    n199 = node-c288() -> ()  [unwired: 2 out]
  }
  n200 = call "goal_loop.vi"("error in"=w9, "Micron config"=w11) -> ("error out"=w4:errorcluster)  [unwired: 9 in]
  n201 = call "manipulator_loop.vi"("error in"=w9, "Micron config"=w11) -> ("error out"=w3:errorcluster)  [unwired: 6 in]
  n202 = call "safety_loop.vi"("error in"=w9, "Micron config"=w11) -> ("error out"=w1:errorcluster)  [unwired: 9 in]
  n203 = call "logger_loop.vi"("error in"=w9, "Micron config"=w11) -> ("error out"=w2:errorcluster)  [unwired: 9 out]
  n204 = call "asap_micron_loop.vi"("ASAP config"=w21, "error in"=w9, "Micron config"=w11) -> ("error out"=w5:errorcluster)  [unwired: 5 out]
  n205 = Merge Errors(w5, w4, w3, w2, w1) -> (w8:errorcluster)
  n206 = Merge Errors(w8, w7) -> (w6:errorcluster)
  n207 = call "cleanup.vi"("error in"=w6, "Configuration"=w21) -> ("error out"=w20:errorcluster)  [unwired: 1 out]
  n208 = node-c288(w23) -> ()  [unwired: 1 out]
  n209 = call "micron_cleanup.vi"("error in"=w20, "Micron config"=w11) -> ("error out"=w25:errorcluster)  [unwired: 9 out]
  n210 = call <vilib>:"Simple Error Handler.vi"("error in (no error)"=w25) -> ()  [unwired: 1 in, 8 out]
  n211 = call "log_watcher.vi"() -> ()  [unwired: 12 in]
  n212 = node-c288(w26) -> (w12:errorcluster)
  n213 = flat-sequence {
    tunnel: w12 -> [w302]
    tunnel: [w302] -> w7
    frame #0 {
      n214 = shared-variable ".\\Micron_rt_vars.lvlib\\Stop"(TRUE ("Stop")) -> ()  [unwired: 2 out]
    }
  }
  n215 = node-c288(w16) -> ()  [unwired: 1 out]
